vi "Strip Template from Base Name.vi"(6 "trim whitespace (T)":bool=TRUE, 8 "error in":errorcluster, 11 "template base name":string) -> (0 "error out":errorcluster, 3 "stripped base name":string)   [LabVIEW 2020, in "Template Tool.lvlib"]
uses:
  Template Tool.lvlib
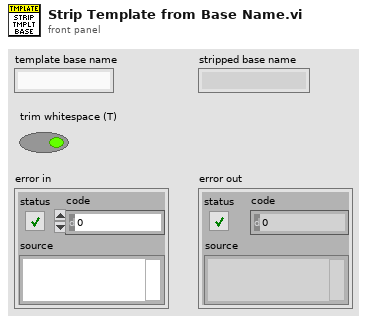
[diagram p1: front panel]
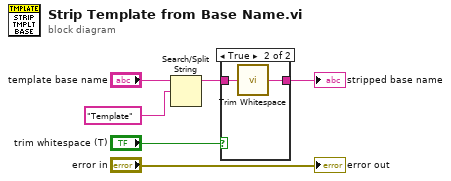
[diagram p0: block diagram]
diagram:
  n1 = Search/Split String(string="template base name", search string/char (-)="Template") -> (substring before match=w5:string)  [unwired: 1 in, 2 out]
  n2 = case shown="True" "trim whitespace (T)" {
    tunnel: w5 -> [w7 w9]
    tunnel: [w7 w8] -> w3
    frame False {
    }
    frame True {
      n3 = call <vilib>:"Trim Whitespace.vi"("string"=w9) -> ("trimmed string"=w8:string)  [unwired: 1 in]
    }
  }
  "stripped base name" <- w3
  "error out" <- "error in"
